vi "SimplerFastCMOSTest.vi"() -> ()   [LabVIEW 2011]
uses:
  CameraConfig.ctl
  BeadTracker2.llb/GenericCameraConfigType.ctl
  qtrk/QTrk.llb/QTrkSettings.ctl
  qtrk/QTrk.llb/QTrkLocalizationType.ctl
  qtrk/QTrk.llb/QTrkZCommandType.ctl
  qtrk/QTrk.llb/QTrkLocalizationResult.ctl
  qtrk/QTrk.llb/QTrkLocalizationJob.ctl
  qtrk/QTrk.llb/XYZf.ctl
  qtrk/QTrk.llb/QTrkPixelDataType.ctl
  qtrk/QTrk.llb/QTrkDLL.vi
panel:
  in  "2D Localization Type":T1=enum."Quadrant Interpolation"
  out "Y":sgl[](graph)
  out "Framerate":i32
  out "Timestamp":u32
  out "X":sgl[](graph)
  in  "Bead index":i32
  in  "Stop result display":bool
  out "Timestamps":u32(graph)
  out "result count":i32
  in  "QTrk Settings":T2={"Image width"=150, "Image height"=150, "Number of threads (CPU based)"=-1, "CUDA Device"=-2, "COM Background correction factor"=0.0, "ZLUT MinRadius"=8.0, "ZLUT Radial sample density"=3.0, "ZLUT Angular sample density"=0.7, "ZLUT ROI Coverage"=0.7, "QI Iterations"=3, "QI MinRadius"=5.0, "QI Radial sample density"=2.5, "QI Angular sample density"=0.7, "QI ROI Coverage"=1.0, "QI Angular Step \nIteration Factor"=1.5, "XCOR Profile Length"=32, "XCOR Profile Width"=2, "XCOR Iterations"=1, "Gaussian 2D Fit Iterations"=6, "Gaussian 2D Sigma (pixels)"=3.0}
  out "FPS":i32
  out "Status Information : Temperature":dbl
  out "Status Information : Frame Count":u32
  out "Status Information : Lost Frames":u32
  out "Last Valid Buffer Index":i32
  in  "Show image":bool
  out "Actual Width":u32
  out "Buffer Number":i32
  out "Image":T3(plugin-control)
  out "total serial timeout count":i16
  out "Initialized?":bool
  in  "stop":bool
  in  "Camera in":T4={"Gain [1-4]"=1.0, "Offset"=1, "Mode"=6, "ROIs"=[{"X"=240, "Y"=100}, {"X"=144, "Y"=610}], "ROI Size"={"X"=200, "Y"=200}, "Number of buffers"=100, "Use hardware multiple-ROI?"=TRUE, "GenericCameraConfig"={"Framerate (Hz)"=300, "Exposure time (us)"=2000, "Image size"={"Width"=1280, "Height"=1024}}}
  out "Acquiring?":bool
  # "-2: Use all devices\n-1: Use best device"
  # "us"
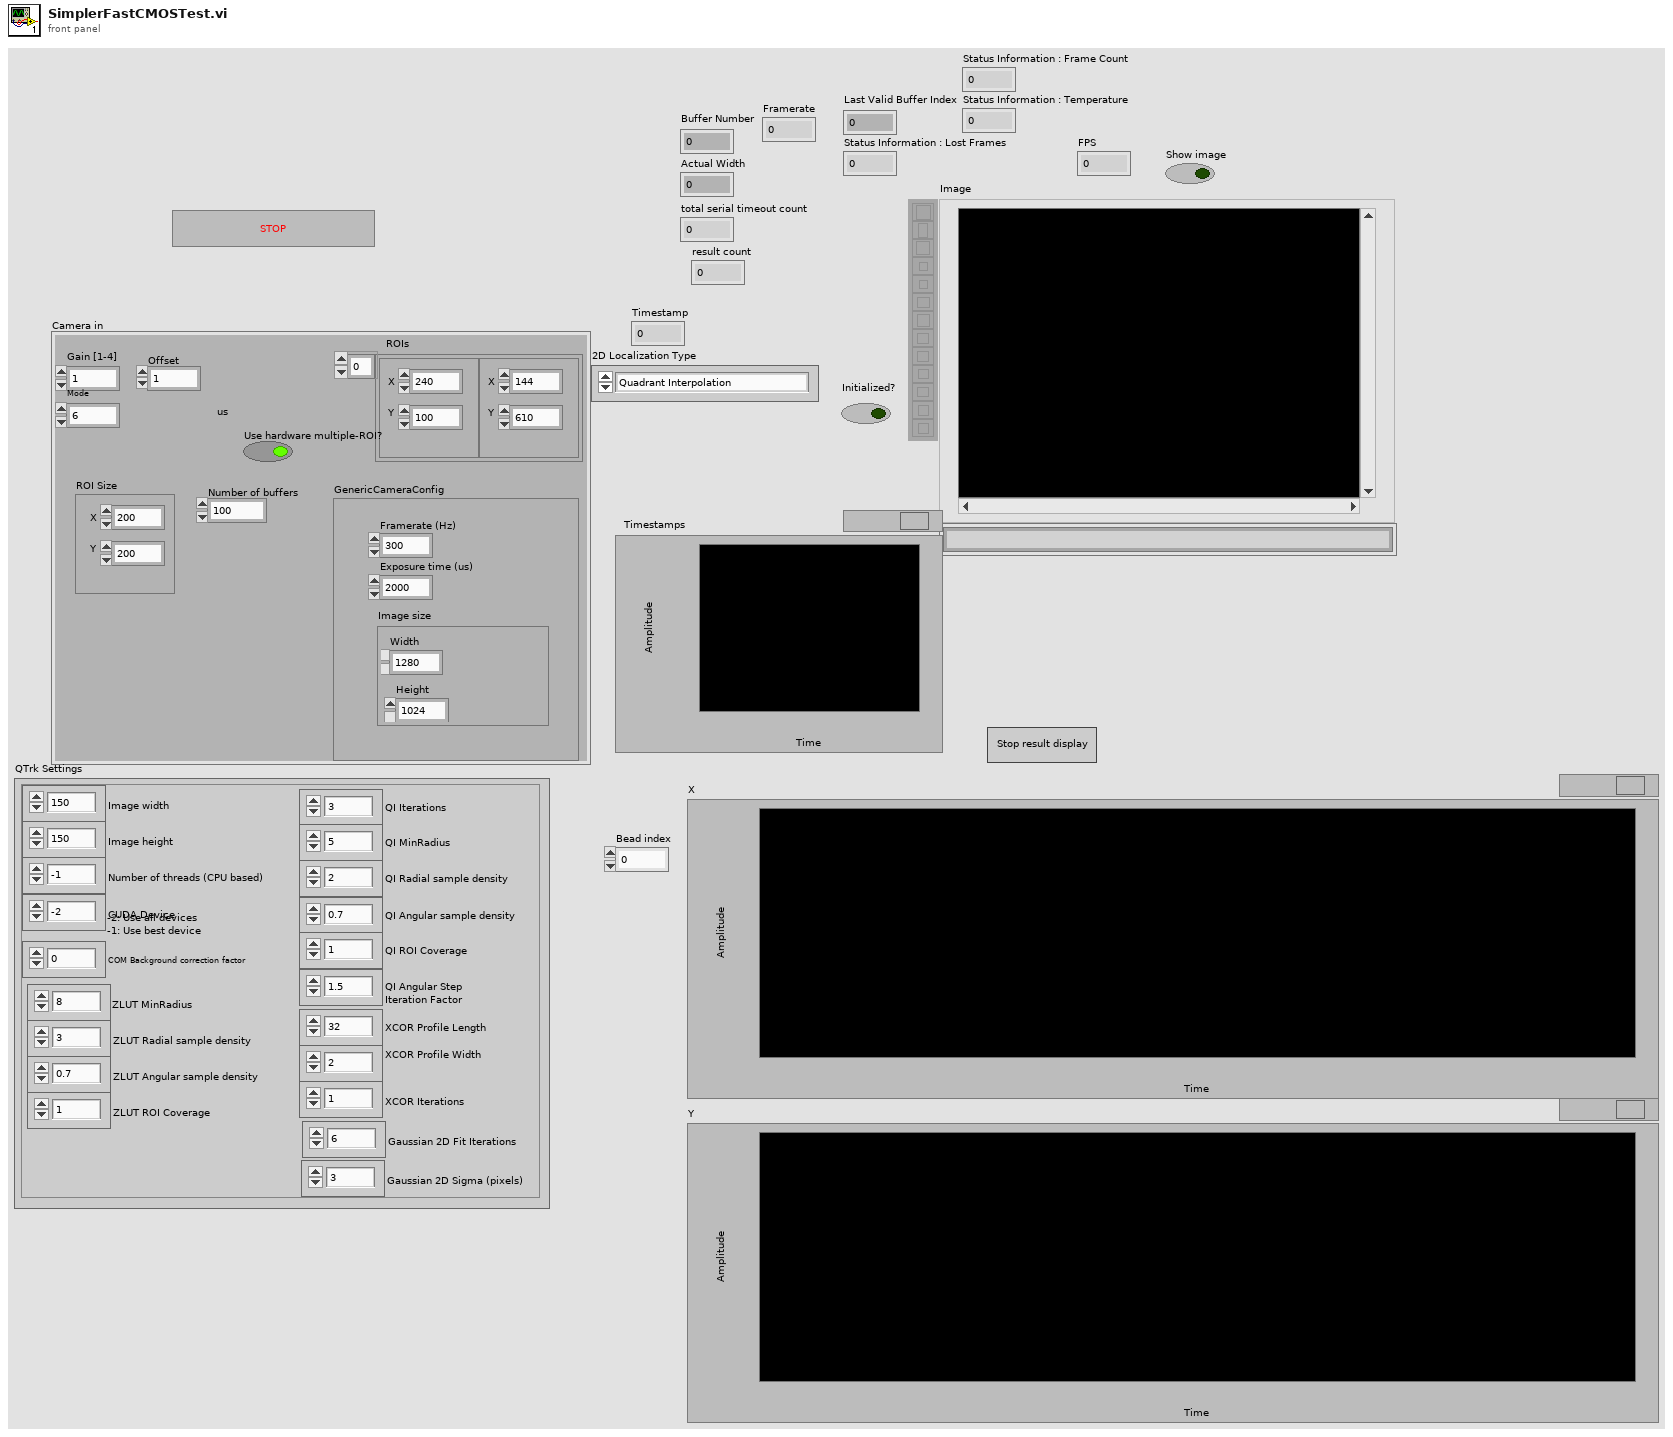
[diagram p1: front panel]
types:
  T1 = typedef "QTrkLocalizationType.ctl" = enum16{"Center-of-Mass", "1D Cross-Correlation", "Quadrant Interpolation", "Gaussian 2D MLE"}
  T2 = typedef "QTrkSettings.ctl" = cluster{"Image width":i32, "Image height":i32, "Number of threads (CPU based)":i32, "CUDA Device":i32, "COM Background correction factor":sgl, "ZLUT MinRadius":sgl, "ZLUT Radial sample density":sgl, "ZLUT Angular sample density":sgl, "ZLUT ROI Coverage":sgl, "QI Iterations":i32, "QI MinRadius":sgl, "QI Radial sample density":sgl, "QI Angular sample density":sgl, "QI ROI Coverage":sgl, "QI Angular Step \nIteration Factor":sgl, "XCOR Profile Length":i32, "XCOR Profile Width":i32, "XCOR Iterations":i32, "Gaussian 2D Fit Iterations":i32, "Gaussian 2D Sigma (pixels)":sgl}
  T3 = typedef "IMAQ Image.ctl" = refnum<image>
  T4 = typedef "CameraConfig.ctl" = cluster{"Gain [1-4]":sgl, "Offset":i16, "Mode":i16, "ROIs":cluster{"X":i32, "Y":i32}[], "ROI Size":cluster{"X":i32, "Y":i32}, "Number of buffers":i32, "Use hardware multiple-ROI?":bool, "GenericCameraConfig":T5}
  T5 = typedef "GenericCameraConfigType.ctl" = cluster{"Framerate (Hz)":i32, "Exposure time (us)":i32, "Image size":cluster{"Width":i32, "Height":i32}}
  T6 = typedef "QTrkLocalizationResult.ctl" = cluster{"Queue Params":T7, "Position":T8, "Fast Estimate Position":cluster{"X":sgl, "Y":sgl}, "Error":i32}
  T7 = typedef "QTrkLocalizationJob.ctl" = cluster{"Frame#":u32, "Timestamp":u32, "ZLUT Index / bead#":i32, "ZLUT Plane":i32, "Initial guess":T8}
  T8 = typedef "XYZf.ctl" = cluster{"X":sgl, "Y":sgl, "Z":sgl}
  T9 = typedef "QTrkZCommandType.ctl" = enum16{"Nothing", "ComputeZ", "BuildRadialZLUT", "BuildImageZLUT", "RadialZLUT+ImageZLUT"}
  T10 = enum16{"Use QTrk settings", "Select best device", "Use all devices", "Use custom list"}
  T11 = typedef "QTrkInstance.ctl" = cluster{"QTrk Pointer":u64}
  T12 = typedef "QTrkPixelDataType.ctl" = enum16{"QTrkU8", "QTrkU16", "QTrkFloat"}
  T13 = enum32{"Map Pixel Pointer", "Unmap Pixel Pointer", "Get Pixels Infos"}
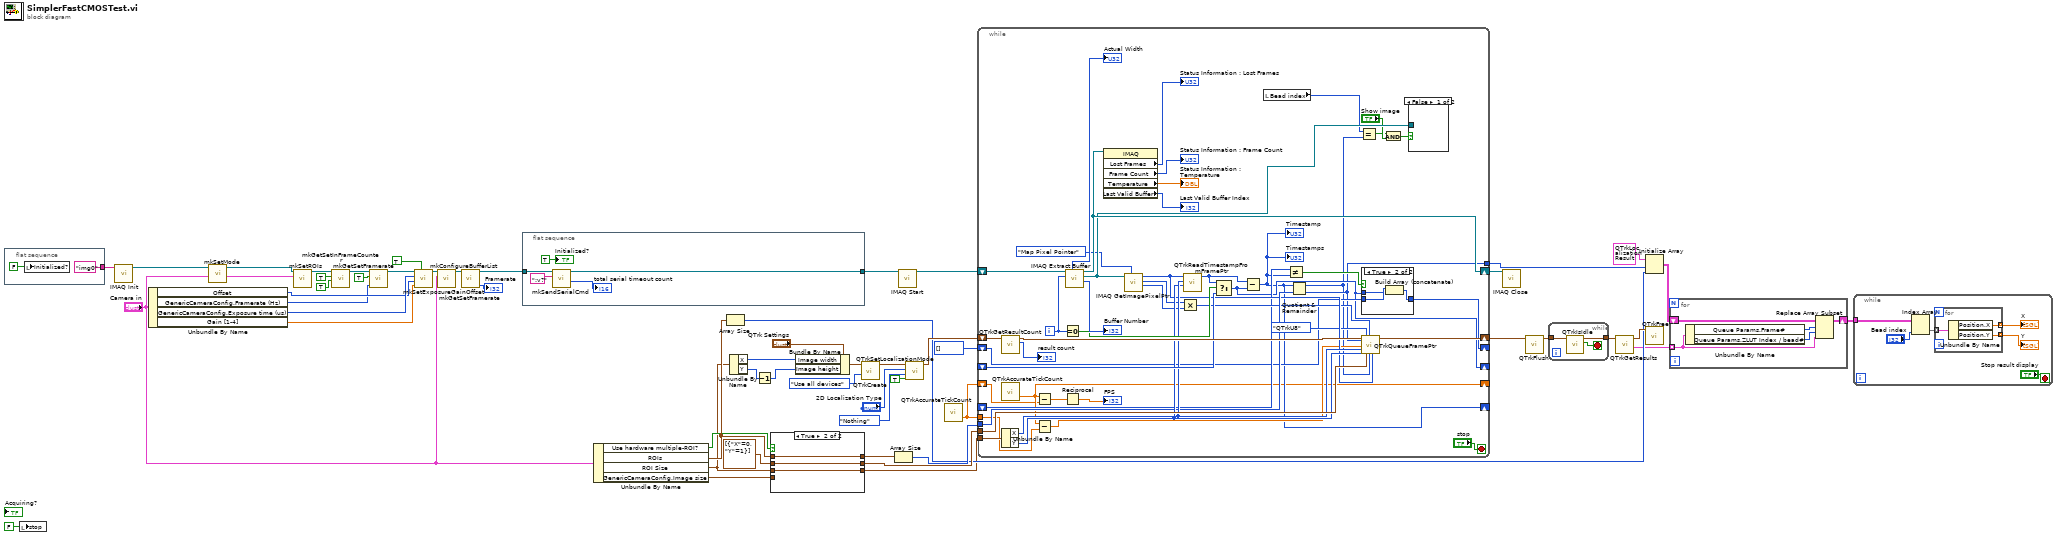
[diagram p0: block diagram]
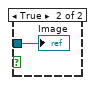
[diagram p4: hidden frame]
diagram:
  n1 = flat-sequence {
    tunnel: ["img0" ("Interface Name")] -> w52
    frame #0 {
      n2 = local write "Initialized?"(FALSE ("Initialized?")) -> ()
    }
  }
  n3 = local write "stop"(FALSE ("stop")) -> ()
  n4 = call <vilib>:"IMAQ Init.vi"("Interface Name"=w52) -> ("IMAQ Session Out"=w11:refnum<k11>)  [unwired: 9 in, 1 out]
  n5 = Unbundle By Name("Camera in") -> ("Offset"=w23:i16, "GenericCameraConfig.Framerate (Hz)"=w18:i32, "GenericCameraConfig.Exposure time (us)"=w24:i32, "Gain [1-4]"=w22:sgl)
  n6 = call "mkSetMode.vi"("Camera in"="Camera in", "IMAQ Refnum in"=w11) -> ("Camera Settings"=w9:T4, "IMAQ Refnum out"=w8:refnum<k11>)  [unwired: 7 in, 1 out]
  n7 = call "mkSetROIs.vi"("Camera in"=w9, "IMAQ Refnum in"=w8) -> ("IMAQ Refnum out"=w25:refnum<k11>)  [unwired: 9 in]
  n8 = call "mkGetSetInFrameCounter.vi"("Set? (F)"=TRUE, "Enable in-frame counter (T)"=TRUE, "IMAQ Refnum in"=w25) -> ("IMAQ Refnum out"=w17:refnum<k11>)  [unwired: 7 in, 1 out]
  n9 = call "mkGetSetFramerate.vi"("Framerate"=w18, "Set? (F)"=TRUE, "IMAQ Refnum out"=w17) -> ("IMAQ Refnum (out)"=w16:refnum<k11>)  [unwired: 5 in, 3 out]
  n10 = call "mkSetExposureGainOffset.vi"("Set? (F)"=TRUE, "Gain [1-4]"=w22, "Offset"=w23, "Exposure time"=w24, "IMAQ Refnum in"=w16) -> ("IMAQ Refnum out"=w15:refnum<k11>)  [unwired: 1 in, 5 out]
  n11 = call "mkConfigureBufferList.vi"("Camera in"="Camera in", "IMAQ Session"=w15) -> ("IMAQ Session (out)"=w13:refnum<k11>)  [unwired: 9 in]
  n12 = call "mkGetSetFramerate.vi"("IMAQ Refnum out"=w13) -> ("Framerate"=→"Framerate":i32, "IMAQ Refnum (out)"=w12:refnum<k11>)  [unwired: 7 in, 2 out]
  n13 = flat-sequence {
    tunnel: [w60] -> w55
    tunnel: w12 -> [w59]
    frame #0 {
      n14 = call "mkSendSerialCmd.vi"("String"=":v?", "IMAQ Refnum in"=w59) -> ("total error count"=→"total serial timeout count":i16, "IMAQ Refnum out"=w60:refnum<k11>)  [unwired: 6 in, 2 out]
      "Initialized?" <- TRUE ("Initialized?")
    }
  }
  n15 = Unbundle By Name("Camera in") -> ("Use hardware multiple-ROI?"=w50:bool, "ROIs"=w36:cluster{"X":i32, "Y":i32}[], "ROI Size"=w4:cluster{"X":i32, "Y":i32}, "GenericCameraConfig.Image size"=w30:cluster{"Width":i32, "Height":i32})
  n16 = Array Size(array=w36) -> (size(s)=w34:i32)
  n17 = Unbundle By Name(w4) -> ("X"=w3:i32, "Y"=w2:i32)
  n18 = Decrement(x=w2) -> (x-1=w1:i32)
  n19 = case shown="True" w50 {
    tunnel: [w66 w69] -> w43
    tunnel: cluster{"X":i32, "Y":i32}[] [{"X"=0, "Y"=1}] ("ROI Positions (corner-based)") -> [w64 w69]
    tunnel: w36 -> [w66 w67]
    tunnel: [w65 w68] -> w29
    tunnel: w30 -> [w65 _]
    tunnel: w4 -> [_ w68]
    tunnel: [w64 w67] -> w7
    frame False {
    }
    frame True {
    }
  }
  n20 = Bundle By Name(cluster="QTrk Settings", "Image width"=w3, "Image height"=w1) -> (w5:T2)
  n21 = call "QTrkCreate.vi"("CUDA device selection"=T10."Use all devices", "QTrk Settings"=w5) -> ("QTrk Instance"=w49:T11)  [unwired: 3 in, 2 out]
  n22 = Array Size(array=w7) -> (size(s)=w42:i32)
  n23 = call <vilib>:"IMAQ Start.vi"("IMAQ Session In"=w55) -> ("IMAQ Session Out"=w53:refnum<k11>)  [unwired: 9 in, 1 out]
  n24 = call "QTrkSetLocalizationMode.vi"("Normalize profile"=TRUE, "Z Command"=QTrkZCommandType."Nothing", "2D Localization Type"="2D Localization Type", "QTrk Instance"=w49) -> ("QTrk Instance"=w48:T11)  [unwired: 7 in]
  n25 = call "QTrkAccurateTickCount.vi"() -> ("seconds"=w41:dbl)  [unwired: 2 in, 1 out]
  n26 = while {
    shift-right: [w109] -> w56
    shift-left: w53 -> [w115]
    shift-right: [w71] -> _
    shift-left: w41 -> [w70]
    shift-right: [w84] -> w39
    shift-left: w48 -> [w105]
    tunnel: w43 -> [w101]
    tunnel: w29 -> [w99]
    shift-right: [w79] -> _
    shift-left: _ -> [w96]
    tunnel: w42 -> [w92]
    tunnel: w41 -> [w86]
    shift-right: [w77] -> _
    shift-left: _ -> [w83]
    shift-right: [w80] -> _
    shift-left: i32[] [] -> [w82]
    tunnel: [w78] -> w35
    i -> [w98]
    stop <- "stop" stop-if-true
    n27 = call "QTrkGetResultCount.vi"("QTrk Instance"=w105) -> ("result count"=→"result count":i32, "QTrk Instance"=w100:T11)  [unwired: 4 in, 1 out]
    n28 = call "QTrkAccurateTickCount.vi"() -> ("seconds"=w71:dbl)  [unwired: 2 in, 1 out]
    n29 = Unbundle By Name(w99) -> ("X"=w94:i32, "Y"=w93:i32)
    n30 = Subtract(x=w71, y=w70) -> (x-y=w108:dbl)
    n31 = Subtract(x=w71, y=w86) -> (x-y=w85:dbl)
    n32 = Equal To 0?(x=w98) -> (x = 0?=w97:bool)
    n33 = Reciprocal(x=w108) -> (1/x=→"FPS":dbl)
    n34 = call <vilib>:"IMAQ Extract Buffer.vi"("Buffer to extract"=w98, "IMAQ Session In"=w115) -> ("Buffer Number"=→"Buffer Number":i32, "Image Out"=w103:T3, "IMAQ Session Out"=w109:refnum<k11>, "Actual Width"=→"Actual Width":u32)  [unwired: 4 in, 2 out]
    n35 = property class="IMAQ"(reference=w109) -> ("Lost Frames"=→"Status Information : Lost Frames":u32, "Frame Count"=→"Status Information : Frame Count":u32, "Temperature"=→"Status Information : Temperature":dbl, "Last Valid Buffer"=→"Last Valid Buffer Index":u32)  [unwired: 1 in, 2 out]
    n36 = call "IMAQ GetImagePixelPtr"("Function"=T13."Map Pixel Pointer", "Image"=w103) -> ("Pixel Size (Bytes)"=w88:i32, "LineWidth(Pixels)"=w89:i32, "Pixel Pointer out"=w91:u64)  [unwired: 4 in, 3 out]
    n37 = Multiply(x=w89, y=w88) -> (x*y=w87:i32)
    n38 = call "QTrkReadTimestampFromFramePtr.vi"("height"=w93, "width"=w94, "imageptr"=w91) -> ("timestamp"=w95:u32)  [unwired: 8 in]
    n39 = Select(t=w95, s=w97, f=w96) -> (s? t:f=w79:u32)
    n40 = Subtract(x=w95, y=w79) -> (x-y=w77:u32)
    "Timestamps" <- w77
    "Timestamp" <- w77
    n41 = local read "Bead index"() -> (w72:i32)
    n42 = Not Equal?(x=w83, y=w77) -> (x != y?=w81:bool)
    n43 = Quotient & Remainder(x=w77, y=w92) -> (x-y*floor(x/y)=w73:u32, floor(x/y)=w78:u32)
    n44 = Equal?(x=w72, y=w73) -> (x = y?=w74:bool)
    n45 = case shown="True" w81 {
      tunnel: w82 -> [w117 w120]
      tunnel: w79 -> [_ w119]
      tunnel: [w117 w118] -> w80
      frame False {
      }
      frame True {
        n46 = Build Array (concatenate)(w120, w119) -> (w118:u32[])
      }
    }
    n47 = call "QTrkQueueFramePtr.vi"("QTrk Instance"=w100, "frame#"=w78, "timestamp"=w85, "width"=w94, "height"=w93, "Pixel data type"=QTrkPixelDataType."QTrkU8", "ROI Positions (corner-based)"=w101, "Image pitch\n(bytes per row)"=w87, "ZLUT Index offset (0)"=w73, "Image Pointer"=w91) -> ("QTrk Instance (out)"=w84:T11)  [unwired: 8 in, 1 out]
    n48 = And(x=w74, y="Show image") -> (x .and. y?=w75:bool)
    n49 = case shown="False" w75 {
      tunnel: w103 -> [_ w121]
      frame False {
      }
      frame True {
        "Image" <- w121
      }
    }
  }
  n50 = call <vilib>:"IMAQ Close.vi"("IMAQ Session In"=w56) -> ()  [unwired: 1 in, 10 out]
  n51 = call "QTrkFlush.vi"("QTrk Instance"=w39) -> ("QTrk Instance (out)"=w28:T11)  [unwired: 9 in, 1 out]
  n52 = while {
    tunnel: w28 -> [w123]
    tunnel: [w122] -> w27
    stop <- w124 stop-if-true
    n53 = call "QTrkIsIdle.vi"("QTrk Instance"=w123) -> ("Currently idle?"=w124:bool, "QTrk Instance (out)"=w122:T11)  [unwired: 8 in, 1 out]
  }
  n54 = call "QTrkGetResults.vi"("QTrk Instance"=w27) -> ("results"=w33:T6[], "QTrk Instance"=w38:T11)  [unwired: 4 in, 1 out]
  n55 = Initialize Array(T6 {"Queue Params"={"Frame#"=0, "Timestamp"=0, "ZLUT Index / bead#"=0, "ZLUT Plane"=0, "Initial guess"={"X"=0.0, "Y"=0.0, "Z"=0.0}}, "Position"={"X"=0.0, "Y"=0.0, "Z"=0.0}, "Fast Estimate Position"={"X"=0.0, "Y"=0.0}, "Error"=0} ("Localization Result"), w35, w34) -> (w32:T6[][])
  n56 = call "QTrkFree.vi"("QTrk Instance"=w38) -> ()  [unwired: 6 in, 1 out]
  n57 = for {
    tunnel: w33 -> [w125] mode=indexing
    shift-right: [w128] -> w31
    shift-left: w32 -> [w129]
    n58 = Unbundle By Name(w125) -> ("Queue Params.Frame#"=w127:u32, "Queue Params.ZLUT Index / bead#"=w126:i32)
    n59 = Replace Array Subset(array=w129, new element=w125, index (row)=w127, index (col)=w126) -> (w128:T6[][])
  }
  n60 = while {
    tunnel: w31 -> [w134]
    stop <- "Stop result display" stop-if-true
    n61 = Index Array(array=w134, index (col)="Bead index") -> (element=w132:T6[])  [unwired: 1 in]
    n62 = for {
      tunnel: w132 -> [w138] mode=indexing
      tunnel: [w137] -> w131 mode=indexing
      tunnel: [w136] -> w130 mode=indexing
      n63 = Unbundle By Name(w138) -> ("Position.X"=w137:sgl, "Position.Y"=w136:sgl)
    }
    "X" <- w131
    "Y" <- w130
  }
